vi "test.vi"() -> ()   [LabVIEW 2022 SP3]
uses:
  <vilib>/Astemes/LUnit/Test Case.lvclass
  <resource>/plugins/PopupMenus/support/Shortcut Menu Item Definition.ctl
  <resource>/plugins/PopupMenus/support/Transaction Control.ctl
  <resource>/plugins/PopupMenus/support/Position In Menu.ctl
  <resource>/plugins/PopupMenus/support/Relative Position.ctl
  <resource>/plugins/PopupMenus/support/Checkmark Status.ctl
  <resource>/plugins/PopupMenus/support/Enabled Menu Item Status.ctl
panel:
  in  "LUnit Test Case In":refnum<class "Test Case.lvclass">
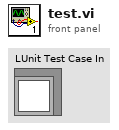
[diagram p1: front panel]
types:
  T1 = typedef "Shortcut Menu Item Definition.ctl" = cluster{"Menu Item Display Name":string, "Menu Item Tag Suffix":string, "Path To Execution VI or MNU":path, "Transaction Control":T2, "Position In Menu":T3, "Checkmark Status":T5, "Enabled Status":T6}
  T2 = typedef "Transaction Control.ctl" = enum8{"LabVIEW auto-wraps execution VI", "Execution VI will define if needed"}
  T3 = typedef "Position In Menu.ctl" = cluster{"Relative":T4, "Existing Item Tag":string}
  T4 = typedef "Relative Position.ctl" = enum8{"Before", "Instead of", "After", "Into Submenu"}
  T5 = typedef "Checkmark Status.ctl" = enum8{"Unchecked", "Checked"}
  T6 = typedef "Enabled Menu Item Status.ctl" = enum8{"Enabled", "Disabled"}
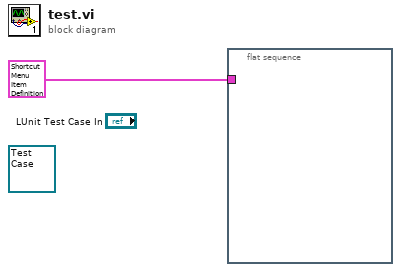
[diagram p0: block diagram]
diagram:
  (unwired) refnum<class "Test Case.lvclass"> refnum ("LUnit Test Case In")
  n1 = flat-sequence {
    tunnel: T1 {"Menu Item Display Name"="", "Menu Item Tag Suffix"="", "Path To Execution VI or MNU"=path "", "Transaction Control"=enum."LabVIEW auto-wraps execution VI", "Position In Menu"={"Relative"=enum."Before", "Existing Item Tag"=""}, "Checkmark Status"=enum."Unchecked", "Enabled Status"=enum."Enabled"} ("Cluster") -> [_]
    frame #0 {
    }
  }
